vi "Calculate Scale.vi"(10 "FoV":dbl, 11 "Image Resolution":i32) -> (3 "Scale":dbl)   [LabVIEW 2012]
panel:
  # "For use with Compute Angle.vi."
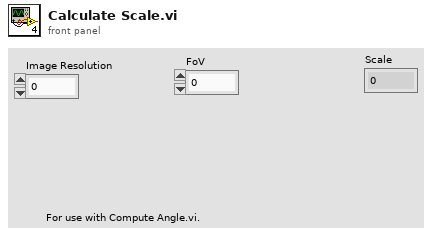
[diagram p1: front panel]
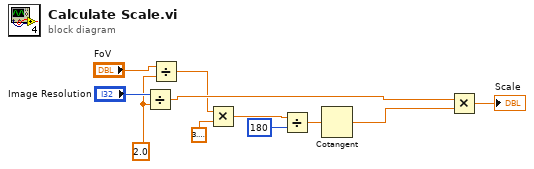
[diagram p0: block diagram]
diagram:
  w2 = 2.0
  n1 = Divide(x="Image Resolution", y=w2) -> (x/y=w9:dbl)
  n2 = Divide(x="FoV", y=w2) -> (x/y=w1:dbl)
  n3 = Multiply(x=w1, y=3.141592653589793) -> (x*y=w7:dbl)
  n4 = Divide(x=w7, y=180) -> (x/y=w6:dbl)
  n5 = Cotangent(1:w6) -> (0:w5:dbl)
  n6 = Multiply(x=w9, y=w5) -> (x*y=→"Scale":dbl)
